vi "manageDependenciesScript_VIs.vi"() -> ()   [LabVIEW 2016]
panel:
  out "Class Name":string
  out "Owner":refnum<vi>
  out "number of replacements":i32
  out "Dependency Paths":path[](array[path])
  out "Dependency Names":string[](array[string])
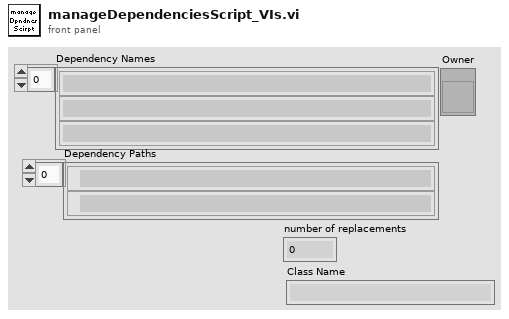
[diagram p1: front panel]
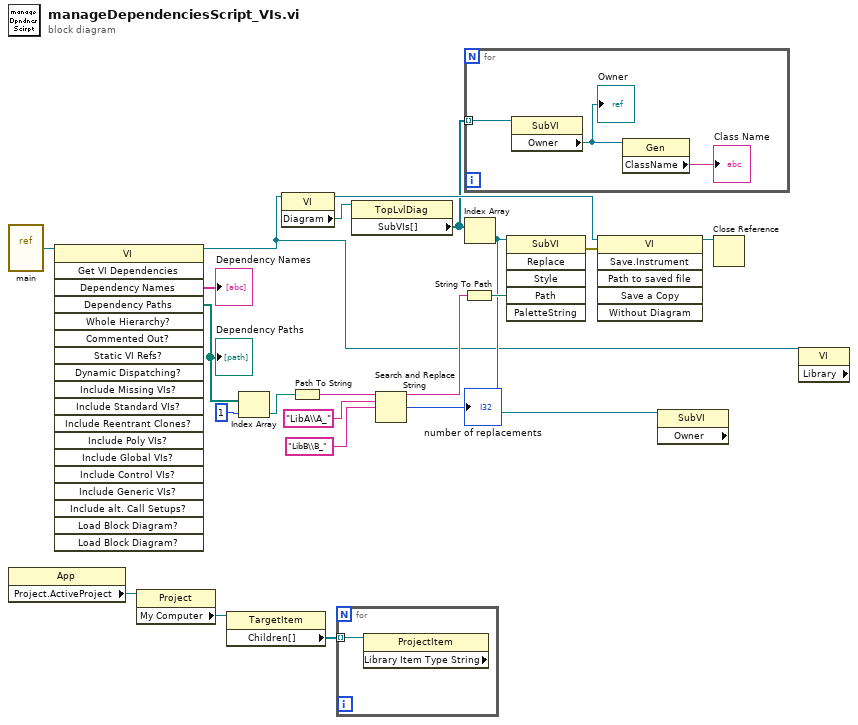
[diagram p0: block diagram]
diagram:
  n1 = vi-ref "main.vi"() -> (w21:refnum<vi>)
  n2 = property class="App"() -> ("Project.ActiveProject"=w5:refnum<vi>)  [unwired: 2 in, 2 out]
  n3 = invoke class="VI" method="Get VI Dependencies"(reference=w21) -> (reference out=w1:refnum<vi>, "Dependency Names"=→"Dependency Names":string[], "Dependency Paths"=w18:path[])  [unwired: 18 in, 16 out]
  "Dependency Paths" <- w18
  n4 = property class="Project"(reference=w5) -> ("My Computer"=w4:refnum<vi>)  [unwired: 1 in, 2 out]
  n5 = property class="TargetItem"(reference=w4) -> ("Children[]"=w3:refnum<vi>[])  [unwired: 1 in, 2 out]
  n6 = Index Array(array=w18, index=1) -> (element=w17:path)
  n7 = property class="VI"(reference=w1) -> (reference out=w13:refnum<vi>, "Diagram"=w19:refnum<vi>)  [unwired: 1 in, 1 out]
  n8 = Path To String(path=w17) -> (string=w16:string)
  n9 = for {
    tunnel: w3 -> [w22] mode=indexing
    n10 = property class="ProjectItem" props=["Library Item Type String"](reference=w22) -> ()  [unwired: 1 in, 3 out]
  }
  n11 = property class="TopLvlDiag"(reference=w19) -> ("SubVIs[]"=w6:refnum<vi>[])  [unwired: 1 in, 2 out]
  n12 = Search and Replace String(input string=w16, search string="LibA\\A_" ("substring (\"\")"), replace string="LibB\\B_" ("replace string (\"\")")) -> (result string=w15:string, number of replacements=→"number of replacements":i32)  [unwired: 5 in, 2 out]
  n13 = String To Path(string=w15) -> (path=w14:path)
  n14 = for {
    tunnel: w6 -> [w25] mode=indexing
    n15 = property class="SubVI"(reference=w25) -> ("Owner"=w24:refnum<vi>)  [unwired: 1 in, 2 out]
    "Owner" <- w24
    n16 = property class="Gen"(reference=w24) -> ("ClassName"=→"Class Name":string)  [unwired: 1 in, 2 out]
  }
  n17 = Index Array(array=w6) -> (element=w2:refnum<vi>)  [unwired: 1 in]
  n18 = invoke class="SubVI" method="Replace"(reference=w2, "Path"=w14) -> (error out=w11:errorcluster)  [unwired: 4 in, 5 out]
  n19 = invoke class="VI" method="Save.Instrument"(reference=w13, error in=w11) -> (reference out=w12:refnum<vi>)  [unwired: 4 in, 5 out]
  n20 = property class="SubVI" props=["Owner"](reference=w2) -> ()  [unwired: 1 in, 3 out]
  n21 = Close Reference(reference=w12) -> ()  [unwired: 1 in, 1 out]
  n22 = property class="VI" props=["Library"](reference=w1) -> ()  [unwired: 1 in, 3 out]
